vi "Is Error.vi"(11 "Base Queue Actor in":refnum<class "Base Queue Actor.lvclass">) -> (3 "Base Queue Actor out":refnum<class "Base Queue Actor.lvclass">)   [LabVIEW 2021, in "jettl.lvlib" / "Base Queue Actor.lvclass"]
uses:
  Base Queue Actor.lvclass
  Queue State/Error Queue State/Error Queue State.lvclass
  C:/git/jettl/src/jettl/Queue State/Queue State/Queue State.lvclass
  Base Queue Actor.lvclass/Base Queue Actor.ctl
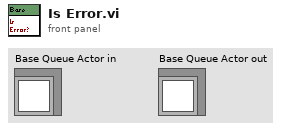
[diagram p1: front panel]
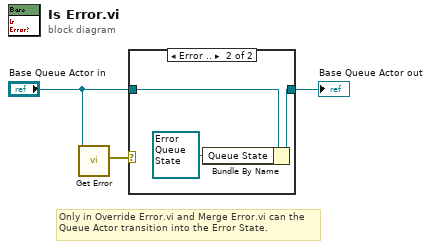
[diagram p0: block diagram]
diagram:
  # "Only in Override Error.vi and Merge Error.vi can the Queue Actor transition into the Error State."
  n1 = call-dynamic "Get Error.vi"("Base Queue Actor in"="Base Queue Actor in") -> ("Error"=w3:errorcluster)  [unwired: 10 in]
  n2 = case shown="Error .." w3 {
    tunnel: [w4 w6] -> w1
    tunnel: "Base Queue Actor in" -> [w4 w7]
    frame No Error {
    }
    frame Error {
      n3 = Bundle By Name(cluster=w7, "Queue State"=refnum<class "Error Queue State.lvclass"> refnum ("jettl.lvlib:jettl Queue Actor.lvlib:Error State.lvclass")) -> (w6:refnum<class "Base Queue Actor.lvclass">)
    }
  }
  "Base Queue Actor out" <- w1
